vi "PH_SRDG645.set i Attr and create DIM services.vi"(0 "i ref in":refnum<vi>, 5 "error in (no error)":errorcluster) -> (14 "i ref out":refnum<vi>, 17 "i Attr":T1={"GUI Refs"={"Delete"=refnum, "Device Errors"=refnum, "Trigger"=refnum, "Default Name"=refnum, "Firmware Revision"=refnum, "Serial Number"=refnum, "Model"=refnum, "Visa resource name"=refnum}, "Service ID Rate"=-1, "Service IDs Channelinfo"=[], "VISA resource name"="", "Device Errors"=[], "Trigger"={"Source"=0, "Rate [Hz]"=1000.0, "Level [V]"=1.0}, "Channels"={"T1"={"Delay [s]"=0.0, "relative to"=0}, "A"={"Delay [s]"=0.0, "relative to"=0}, "B"={"Delay [s]"=0.0, "relative to"=0}, "C"={"Delay [s]"=0.0, "relative to"=0}, "D"={"Delay [s]"=0.0, "relative to"=0}, "E"={"Delay [s]"=0.0, "relative to"=0}, "F"={"Delay [s]"=0.0, "relative to"=0}, "G"={"Delay [s]"=0.0, "relative to"=0}, "H"={"Delay [s]"=0.0, "relative to"=0}}, "GUI Refs Channels"=[], "Outputs"={"AB"={"Level Offset [V]"=0.0, "Amplitue [V]"=0.0, "Polarity"=0}, "CD"={"Level Offset [V]"=0.0, "Amplitue [V]"=0.0, "Polarity"=0}, "EF"={"Level Offset [V]"=0.0, "Amplitue [V]"=0.0, "Polarity"=0}, "GH"={"Level Offset [V]"=0.0, "Amplitue [V]"=0.0, "Polarity"=0}, "T0"={"Level Offset [V]"=0.0, "Amplitue [V]"=0.0, "Polarity"=0}}, "GUI Refs Outputs"=[], "Serial Number"="", "Firmweare Revision"="", "Model"=""} {"Outputs"."T0"."Polarity" items=["negative", "positive"]; "Outputs"."GH"."Polarity" items=["negative", "positive"]; "Outputs"."EF"."Polarity" items=["negative", "positive"]; "Outputs"."CD"."Polarity" items=["negative", "positive"]; "Outputs"."AB"."Polarity" items=["negative", "positive"]; "Channels"."H"."relative to" items=["T0", "T1", "A", "B", "C", "D", "E", "F", "G", "H"]; "Channels"."H"."Delay [s]" format="%#_12p"; "Channels"."G"."relative to" items=["T0", "T1", "A", "B", "C", "D", "E", "F", "G", "H"]; "Channels"."G"."Delay [s]" format="%#_12p"; "Channels"."F"."relative to" items=["T0", "T1", "A", "B", "C", "D", "E", "F", "G", "H"]; "Channels"."F"."Delay [s]" format="%#_12p"; "Channels"."E"."relative to" items=["T0", "T1", "A", "B", "C", "D", "E", "F", "G", "H"]; "Channels"."E"."Delay [s]" format="%#_12p"; "Channels"."D"."relative to" items=["T0", "T1", "A", "B", "C", "D", "E", "F", "G", "H"]; "Channels"."D"."Delay [s]" format="%#_12p"; "Channels"."C"."relative to" items=["T0", "T1", "A", "B", "C", "D", "E", "F", "G", "H"]; "Channels"."C"."Delay [s]" format="%#_12p"; "Channels"."B"."relative to" items=["T0", "T1", "A", "B", "C", "D", "E", "F", "G", "H"]; "Channels"."B"."Delay [s]" format="%#_12p"; "Channels"."A"."relative to" items=["T0", "T1", "A", "B", "C", "D", "E", "F", "G", "H"]; "Channels"."A"."Delay [s]" format="%#_12p"; "Channels"."T1"."relative to" items=["T0", "T1", "A", "B", "C", "D", "E", "F", "G", "H"]; "Channels"."T1"."Delay [s]" format="%#_12p"; "Trigger"."Rate [Hz]" format="%#_9p"; "Trigger"."Source" items=["Internal", "External rising edge", "External falling edge", "Single shot external rising edges", "Single shot external falling edges", "Single shot", "Line"]}, 19 "error out":errorcluster)   [LabVIEW 2014, in "PH_SRDG645.lvlib"]
doc: "This VI opens several services to provide instance information."
uses:
  PH_SRDG645.lvlib
  PH_SRDG645.i attribute.ctl
  PH_SRDG645.Trigger.ctl
  PH_SRDG645.Channel Settings.ctl
  PH_Basics/PH_Common/PH_Common.lvlib
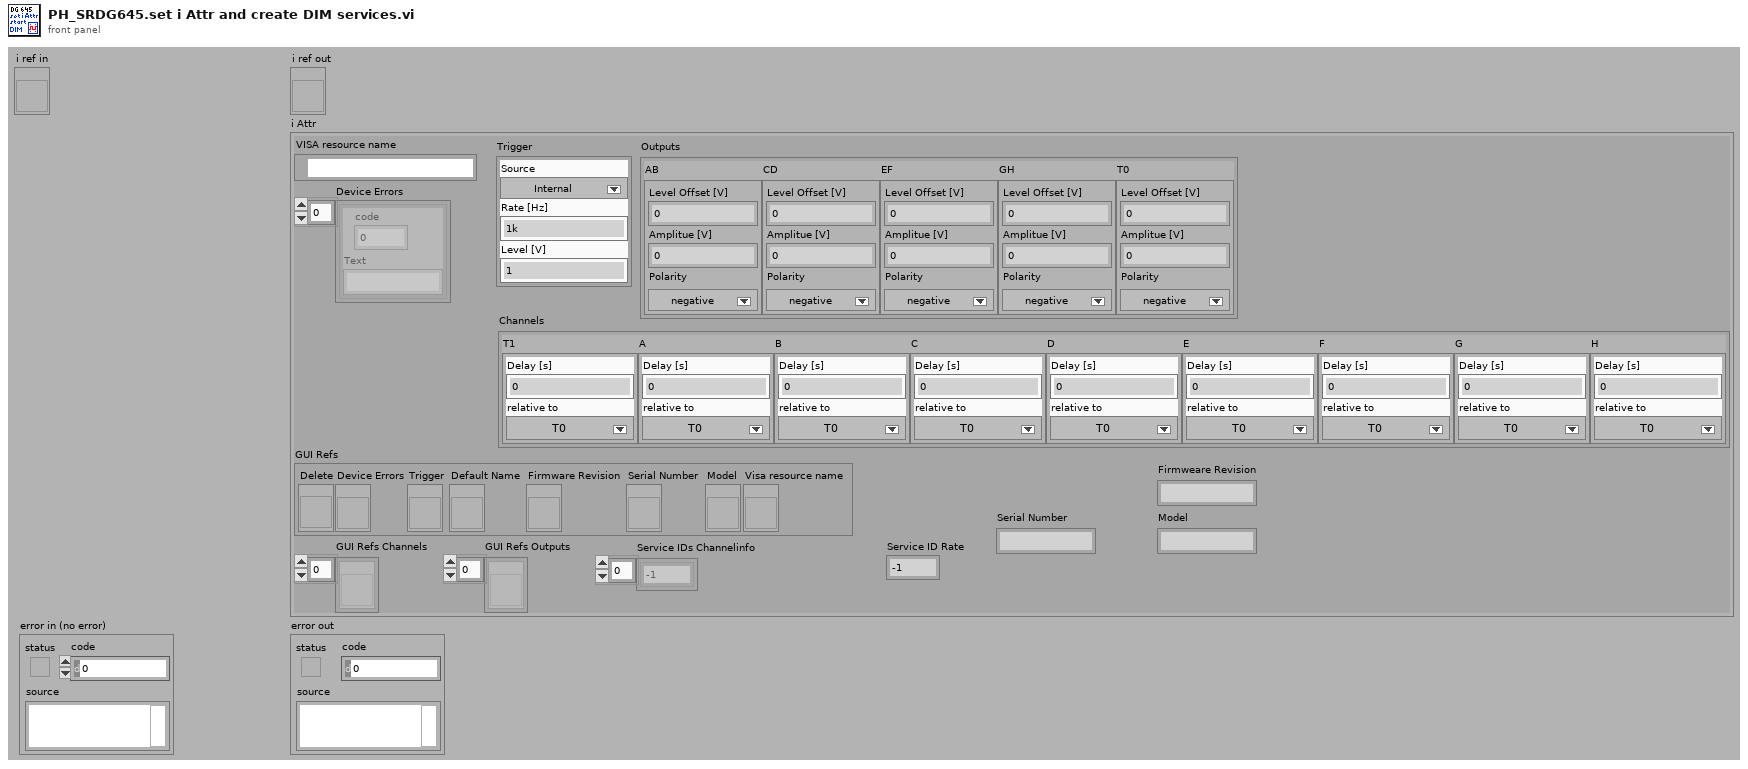
[diagram p1: front panel]
types:
  T1 = typedef "PH_SRDG645.lvlib/PH_SRDG645.i attribute.ctl" = cluster{"GUI Refs":cluster{"Delete":refnum<vi>, "Device Errors":refnum<vi>, "Trigger":refnum<vi>, "Default Name":refnum<vi>, "Firmware Revision":refnum<vi>, "Serial Number":refnum<vi>, "Model":refnum<vi>, "Visa resource name":refnum<vi>}, "Service ID Rate":i32, "Service IDs Channelinfo":i32[], "VISA resource name":refnum<visa-resource-name>, "Device Errors":cluster{"code":i32, "Text":string}[], "Trigger":T2, "Channels":cluster{"T1":T3, "A":T3, "B":T3, "C":T3, "D":T3, "E":T3, "F":T3, "G":T3, "H":T3}, "GUI Refs Channels":refnum<vi>[], "Outputs":cluster{"AB":cluster{"Level Offset [V]":dbl, "Amplitue [V]":dbl, "Polarity":i32}, "CD":cluster{"Level Offset [V]":dbl, "Amplitue [V]":dbl, "Polarity":i32}, "EF":cluster{"Level Offset [V]":dbl, "Amplitue [V]":dbl, "Polarity":i32}, "GH":cluster{"Level Offset [V]":dbl, "Amplitue [V]":dbl, "Polarity":i32}, "T0":cluster{"Level Offset [V]":dbl, "Amplitue [V]":dbl, "Polarity":i32}}, "GUI Refs Outputs":refnum<vi>[], "Serial Number":string, "Firmweare Revision":string, "Model":string}
  T2 = typedef "PH_SRDG645.lvlib/PH_SRDG645.Trigger.ctl" = cluster{"Source":i32, "Rate [Hz]":dbl, "Level [V]":dbl}
  T3 = typedef "PH_SRDG645.lvlib/PH_SRDG645.Channel Settings.ctl" = cluster{"Delay [s]":dbl, "relative to":i32}
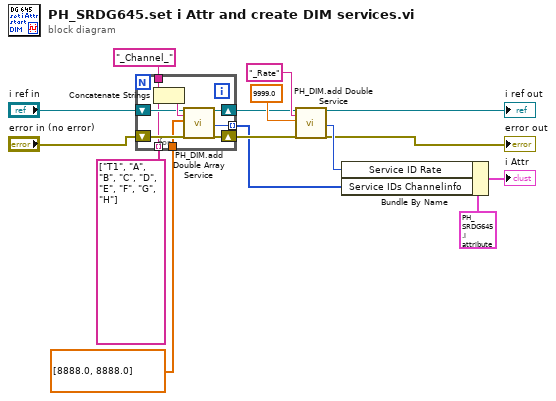
[diagram p0: block diagram]
diagram:
  n1 = for {
    shift-right: [w24] -> w8
    shift-left: "i ref in" -> [w20]
    shift-right: [w22] -> w6
    shift-left: "error in (no error)" -> [w23]
    tunnel: string[] ["T1", "A", "B", "C", "D", "E", "F", "G", "H"] -> [w19] mode=indexing
    tunnel: [w18] -> w5 mode=indexing
    tunnel: dbl[] [8888.0, 8888.0] ("Double Value Array") -> [w17]
    tunnel: "_Channel_" ("string") -> [w16]
    n2 = Concatenate Strings(w16, w19) -> (w21:string)
    n3 = call "PH_DIM.add Double Array Service.vi"("i ref in"=w20, "Service Name"=w21, "Double Value Array"=w17, "error in (no error)"=w23) -> ("i ref out"=w24:refnum<vi>, "Service ID"=w18:i32, "error out"=w22:errorcluster)  [unwired: 13 in]
  }
  n4 = call "PH_DIM.add Double Service.vi"("i ref in"=w8, "Service Name"="_Rate" ("string"), "Double Value"=9999.0, "error in (no error)"=w6) -> ("i ref out"=→"i ref out":refnum<vi>, "Service ID"=w13:i32, "error out"=→"error out":errorcluster)  [unwired: 13 in]
  n5 = Bundle By Name(cluster=T1 {"GUI Refs"={"Delete"=refnum, "Device Errors"=refnum, "Trigger"=refnum, "Default Name"=refnum, "Firmware Revision"=refnum, "Serial Number"=refnum, "Model"=refnum, "Visa resource name"=refnum}, "Service ID Rate"=0, "Service IDs Channelinfo"=[], "VISA resource name"="", "Device Errors"=[], "Trigger"={"Source"=0, "Rate [Hz]"=0.0, "Level [V]"=0.0}, "Channels"={"T1"={"Delay [s]"=0.0, "relative to"=0}, "A"={"Delay [s]"=0.0, "relative to"=0}, "B"={"Delay [s]"=0.0, "relative to"=0}, "C"={"Delay [s]"=0.0, "relative to"=0}, "D"={"Delay [s]"=0.0, "relative to"=0}, "E"={"Delay [s]"=0.0, "relative to"=0}, "F"={"Delay [s]"=0.0, "relative to"=0}, "G"={"Delay [s]"=0.0, "relative to"=0}, "H"={"Delay [s]"=0.0, "relative to"=0}}, "GUI Refs Channels"=[], "Outputs"={"AB"={"Level Offset [V]"=0.0, "Amplitue [V]"=0.0, "Polarity"=0}, "CD"={"Level Offset [V]"=0.0, "Amplitue [V]"=0.0, "Polarity"=0}, "EF"={"Level Offset [V]"=0.0, "Amplitue [V]"=0.0, "Polarity"=0}, "GH"={"Level Offset [V]"=0.0, "Amplitue [V]"=0.0, "Polarity"=0}, "T0"={"Level Offset [V]"=0.0, "Amplitue [V]"=0.0, "Polarity"=0}}, "GUI Refs Outputs"=[], "Serial Number"="", "Firmweare Revision"="", "Model"=""} ("i Attr"), "Service ID Rate"=w13, "Service IDs Channelinfo"=w5) -> (→"i Attr":T1)
